vi "mht2image.vi"(6 "size":i32=60000, 7 "IMGPath":path, 8 "Error in":errorcluster caption="Error in (no error)", 11 "mht":path) -> (0 "Error out":errorcluster, 3 "IMGPath out":path, 5 "ImagePath":path)   [LabVIEW 2016]
uses:
  <vilib>/NI/Tools/String/Tools_String.lvlib
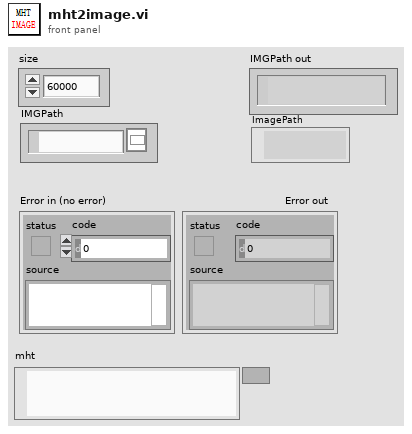
[diagram p1: front panel]
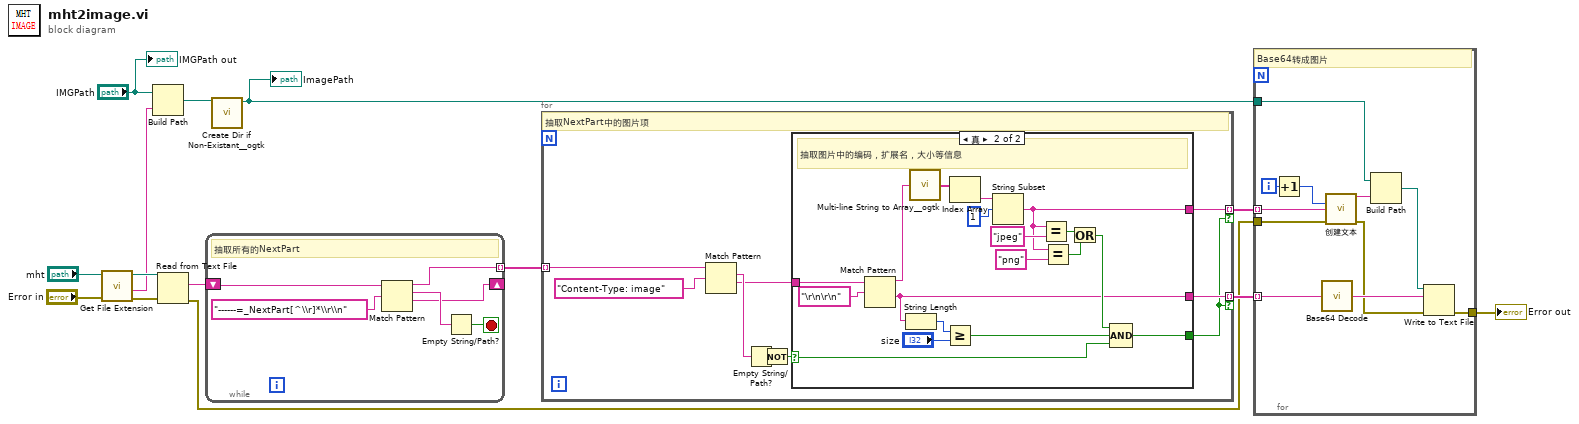
[diagram p0: block diagram]
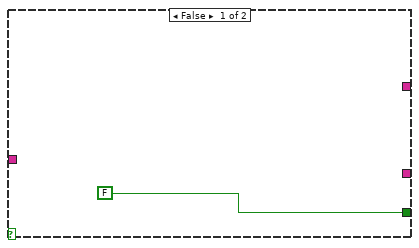
[diagram p2: hidden frame]
diagram:
  n1 = call <vilib>:"Get File Extension.vi"("error in (no error)"="Error in", "file"="mht") -> ("error out"=w9:errorcluster, "filename without extension"=w8:string, "dup file"=w10:path)  [unwired: 5 in, 2 out]
  n2 = Build Path(base path="IMGPath", name or relative path=w8) -> (appended path=w6:path)
  n3 = Read from Text File(file (use dialog)=w10, error in=w9) -> (text=w14:string, error out=w4:errorcluster)  [unwired: 2 in, 2 out]
  n4 = while {
    shift-right: [w15] -> _
    shift-left: w14 -> [w20]
    tunnel: [w16] -> w13 mode=indexing
    stop <- w17 stop-if-true
    # "抽取所有的NextPart"
    n5 = Match Pattern(string=w20, regular expression="------=_NextPart[^\\r]*\\r\\n" ("搜索字符串/字符(-)")) -> (before substring=w16:string, match substring=w18:string, after substring=w15:string)  [unwired: 1 in, 1 out]
    n6 = Empty String/Path?(string/path=w18) -> (empty?=w17:bool)
  }
  n7 = call <userlib>:"Create Dir if Non-Existant__ogtk.vi"("Directory Path"=w6) -> ("dup Directory Path"=w5:path)  [unwired: 8 in, 2 out]
  "ImagePath" <- w5
  n8 = for {
    tunnel: w13 -> [w29] mode=indexing
    tunnel: [w24] -> w11 mode=indexing if=w21
    tunnel: [w22] -> w12 mode=indexing if=w21
    # "抽取NextPart中的图片项"
    n9 = Match Pattern(string=w29, regular expression="Content-Type: image" ("正则表达式")) -> (match substring=w27:string, after substring=w25:string)  [unwired: 1 in, 2 out]
    n10 = Empty String/Path?(string/path=w27) -> (empty?=w26:bool)
    n11 = Not(x=w26) -> (.not. x?=w23:bool)
    n12 = case shown="真" w23 {
      selector: w23 -> [_ w36]
      tunnel: w25 -> [_ w48]
      tunnel: [_ w33] -> w24
      tunnel: [FALSE w37] -> w21
      tunnel: [_ w31] -> w22
      frame False {
      }
      frame True {
        # "抽取图片中的编码，扩展名，大小等信息"
        n13 = Match Pattern(string=w48, regular expression="\r\n\r\n" ("正则表达式")) -> (before substring=w45:string, after substring=w33:string)  [unwired: 1 in, 2 out]
        n14 = String Length(string=w33) -> (length=w32:i32)
        n15 = call <userlib>:"Multi-line String to Array__ogtk.vi"("string"=w45) -> ("lines"=w44:string[])
        n16 = Greater Or Equal?(x=w32, y="size") -> (x >= y?=w35:bool)
        n17 = Index Array(array=w44) -> (element=w43:string)  [unwired: 1 in]
        n18 = String Subset(string=w43, offset (0)=1 ("长度（剩余）")) -> (substring=w31:string)  [unwired: 1 in]
        n19 = Equal?(x=w31, y="jpeg") -> (x = y?=w39:bool)
        n20 = Equal?(x=w31, y="png") -> (x = y?=w38:bool)
        n21 = Or(x=w39, y=w38) -> (x .or. y?=w34:bool)
        n22 = Compound Arithmetic op=AND ("复合运算")(w34, w35, w36) -> (w37:bool)
      }
    }
  }
  n23 = for {
    tunnel: w12 -> [w59] mode=indexing
    tunnel: w11 -> [w56] mode=indexing
    tunnel: w5 -> [w54]
    tunnel: w4 -> [w51]
    tunnel: [w50] -> w1
    i -> [w58]
    # "Base64转成图片"
    n24 = Increment(x=w58) -> (x+1=w49:i32)
    n25 = call <vilib>:"Base64 Decode.vi"("base64 string"=w56) -> ("normal string"=w57:string)
    n26 = call "创建文本"("idx"=w49, "extname"=w59, "error in (no error)"=w51) -> ("Result"=w55:string, "error out"=w52:errorcluster)  [unwired: 11 in]
    n27 = Build Path(base path=w54, name or relative path=w55) -> (appended path=w53:path)
    n28 = Write to Text File(file (use dialog)=w53, text=w57, error in=w52) -> (error out=w50:errorcluster)  [unwired: 1 in, 2 out]
  }
  "Error out" <- w1
  "IMGPath out" <- "IMGPath"
